vi "ZMQ.Handle Error.vi"(8 "error in (no error)":errorcluster, 11 "RemoteControl.ZMQ in":refnum<class "RemoteControl.ZMQ.lvclass">) -> (0 "error out":errorcluster, 3 "RemoteControl.ZMQ out":refnum<class "RemoteControl.ZMQ.lvclass">)   [LabVIEW 2019, in "RemoteControl.ZMQ.lvlib" / "RemoteControl.ZMQ.lvclass"]
uses:
  RemoteControl.ZMQ.lvclass
  <vilib>/addons/zeromq/zmq_socket.lvclass
  <vilib>/addons/zeromq/zeromq.lvlib
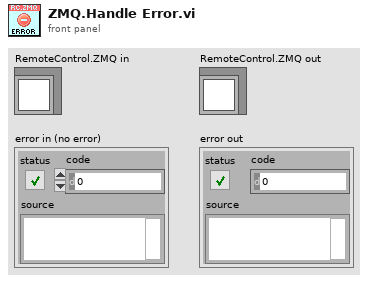
[diagram p1: front panel]
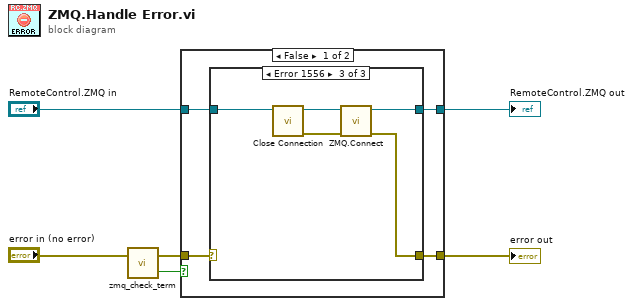
[diagram p0: block diagram]
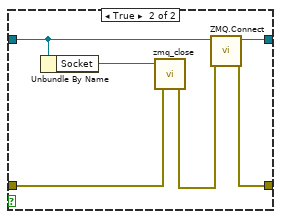
[diagram p4: hidden frame]
diagram:
  n1 = call <vilib>:"zmq_check_term.vi"("error in"="error in (no error)") -> ("term?"=w2:bool, "error out"=w1:errorcluster)  [unwired: 1 in]
  n2 = case shown="False" w2 {
    tunnel: w1 -> [w10 w25]
    tunnel: "RemoteControl.ZMQ in" -> [w7 w21]
    tunnel: [w8 w24] -> w5
    tunnel: [w9 w22] -> w6
    frame False {
      n3 = case shown="Error 1556" w10 {
        selector: w10 -> [w12 w13 _]
        tunnel: [w12 w13 w15] -> w9
        tunnel: [w11 w14 w16] -> w8
        tunnel: w7 -> [w11 w14 w19]
        frame No Error {
        }
        frame Default {
        }
        frame Error {
          n4 = call-dynamic "Close Connection.vi"("RemoteControl.ZMQ in"=w19) -> ("error out"=w17:errorcluster, "RemoteControl.ZMQ out"=w18:refnum<class "RemoteControl.ZMQ.lvclass">)  [unwired: 9 in]
          n5 = call "ZMQ.Connect.vi"("error in (no error)"=w17, "RemoteControl.ZMQ in"=w18) -> ("error out"=w15:errorcluster, "RemoteControl.ZMQ out"=w16:refnum<class "RemoteControl.ZMQ.lvclass">)  [unwired: 8 in]
        }
      }
    }
    frame True {
      n6 = Unbundle By Name(w21) -> ("Socket"=w20:refnum<class "zmq_socket.lvclass">)
      n7 = call <vilib>:"zmq_close.vi"("error in"=w25, "socket"=w20) -> ("error out"=w23:errorcluster)  [unwired: 3 in]
      n8 = call "ZMQ.Connect.vi"("error in (no error)"=w23, "RemoteControl.ZMQ in"=w21) -> ("error out"=w22:errorcluster, "RemoteControl.ZMQ out"=w24:refnum<class "RemoteControl.ZMQ.lvclass">)  [unwired: 8 in]
    }
  }
  "error out" <- w6
  "RemoteControl.ZMQ out" <- w5
